vi "Find Control Index in ConPane.vi"(8 "error in (no error)":errorcluster, 10 "Control Ref":refnum<vi>, 11 "ConPane ref":refnum<vi>) -> (0 "error out":errorcluster, 1 "Found ?":bool, 2 "Terminal index":i32, 3 "ConPane ref Dup":refnum<vi>)   [LabVIEW 2012, in "Scripting Tools.lvlib"]
doc: "Return ConPane Index of on Control if Find.\nDeveloper : Eric Bobillier\nCompagny : Inra\nCreation date : 15/06/2011"
uses:
  Scripting Tools.lvlib
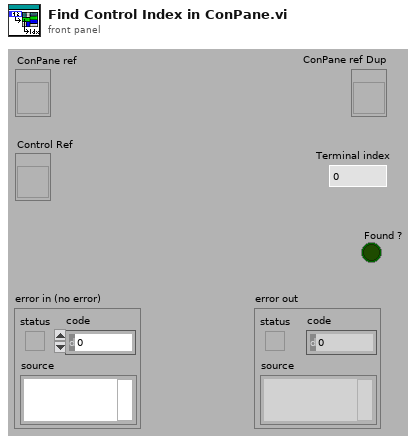
[diagram p1: front panel]
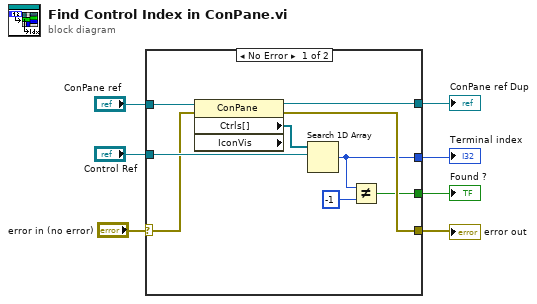
[diagram p0: block diagram]
diagram:
  n1 = case shown="No Error" "error in (no error)" {
    selector: "error in (no error)" -> [w13 w19]
    tunnel: [w11 w19] -> w7
    tunnel: "ConPane ref" -> [w15 w17]
    tunnel: "Control Ref" -> [w14 _]
    tunnel: [w10 w17] -> w3
    tunnel: [w9 _] -> w2
    tunnel: [w8 -1 ("index of element")] -> w1
    frame No Error {
      n2 = property class="ConPane" props=["Ctrls[]", "IconVis"](reference=w15, error in=w13) -> (reference out=w10:refnum<vi>, error out=w11:errorcluster, "Ctrls[]"=w16:refnum<vi>[])  [unwired: 1 out]
      n3 = Search 1D Array(1D array=w16, element=w14) -> (index of element=w8:i32)  [unwired: 1 out]
      n4 = Not Equal?(x=w8, y=-1 ("indice de l'élément")) -> (x != y?=w9:bool)
    }
    frame Error {
    }
  }
  "error out" <- w7
  "ConPane ref Dup" <- w3
  "Found ?" <- w2
  "Terminal index" <- w1
